vi "Daqmx Test VI.vi"() -> ()   [LabVIEW 2018]
uses:
  <vilib>/nisyscfg/Resource Expert Info.ctl
  <resource>/objmgr/daqmx.rc
  <vilib>/nisyscfg/nisyscfg.lvlib
  <resource>/objmgr/nicriosae.rc
panel:
  out "Array 3":string[](array[string])
  out "Array 2":string[](array[string])
  out "Experts":T1[][](array[typedef])
  out "Array":string[](array[string])
  out "Session out 2":refnum<k21> caption="Session out"
  out "Detected Systems":string[](array[string])
  out "DO.NumLines":u32
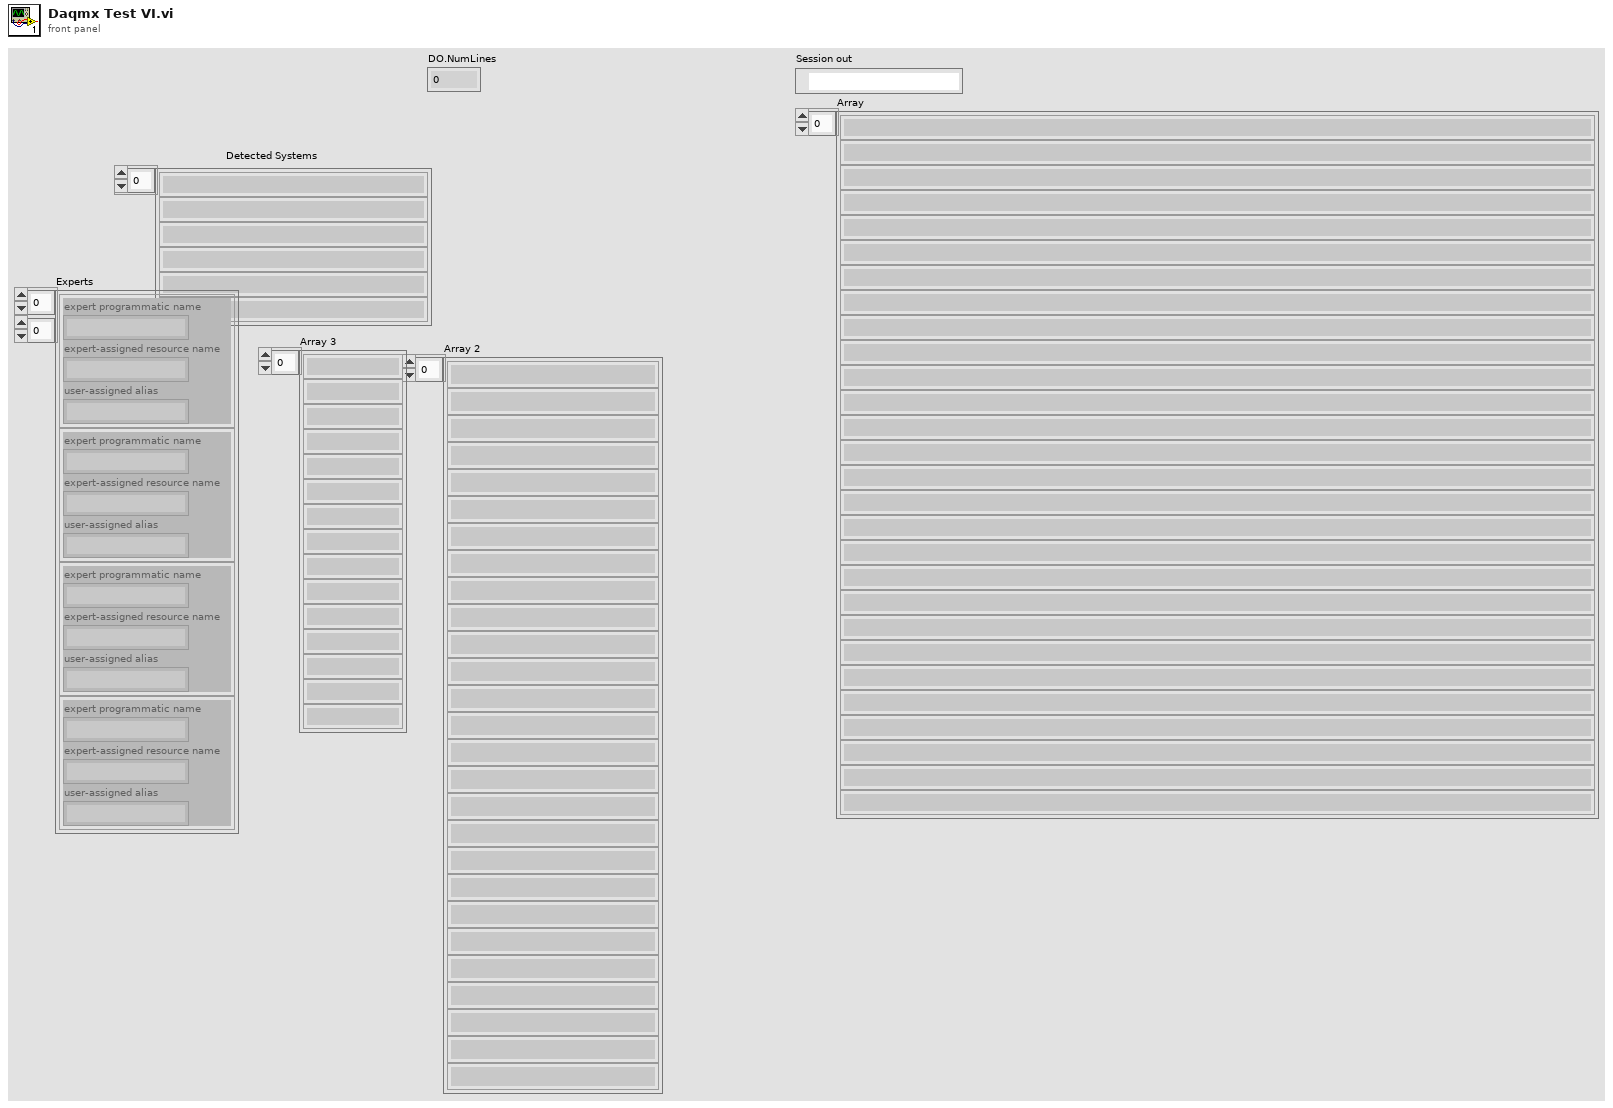
[diagram p1: front panel]
types:
  T1 = typedef "nisyscfg.lvlib/Resource Expert Info.ctl" = cluster{"expert programmatic name":string, "expert-assigned resource name":string, "user-assigned alias":string}
  T2 = typedef "Resource Expert Info.ctl" = cluster{"expert programmatic name":string, "expert-assigned resource name":string, "user-assigned alias":string}
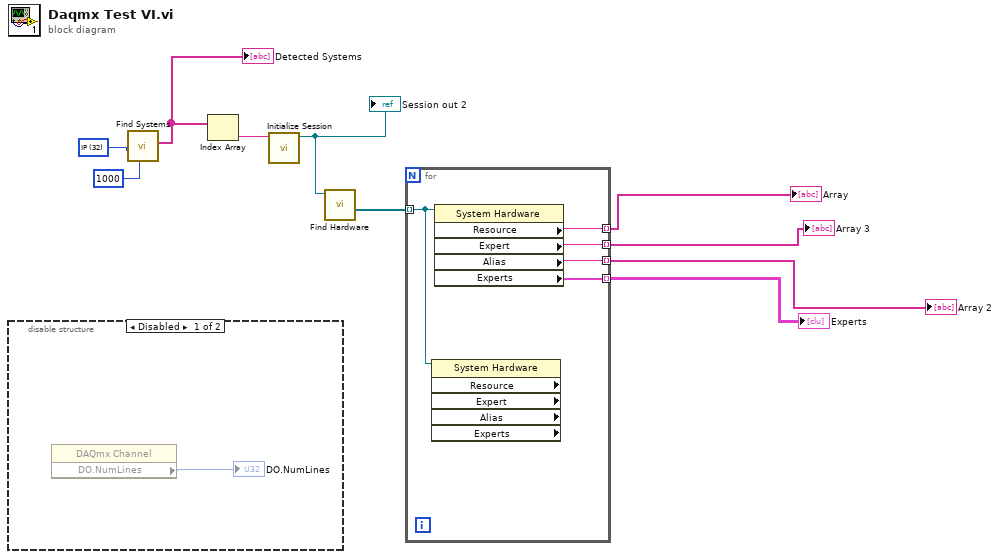
[diagram p0: block diagram]
diagram:
  w9 = u32 32 items=["Hostname"=16, "Hostname (IP)"=18, "Hostname (MAC)"=19, "IP"=32, "IP (Hostname)"=33, "IP (MAC)"=35, "MAC"=48, "MAC (Hostname)"=49, "MAC (IP)"=50] ("Output (Hostname and IP)")
  n1 = disable-structure shown="Disabled" {
    frame Disabled {
      n2 = property class="DAQmx Channel"() -> ("DO.NumLines"=→"DO.NumLines":u32)  [unwired: 2 in, 2 out]
    }
    frame Enabled {
    }
  }
  n3 = call <vilib>:"Find Systems.vi"("Timeout (4000 ms)"=u32 1000, "Output (Hostname and IP)"=w9) -> ("Detected Systems"=w8:string[])  [unwired: 7 in, 2 out]
  "Detected Systems" <- w8
  n4 = Index Array(array=w8) -> (element=w7:string)  [unwired: 1 in]
  n5 = call <vilib>:"Initialize Session.vi"("Target (localhost)"=w7) -> ("Session out"=w6:refnum<k21>)  [unwired: 9 in, 1 out]
  "Session out 2" <- w6
  n6 = call <vilib>:"Find Hardware.vi"("Session in"=w6) -> ("Resources out"=w5:refnum<k20>[])  [unwired: 7 in, 3 out]
  n7 = for {
    tunnel: w5 -> [w12] mode=indexing
    tunnel: [w16] -> w4 mode=indexing
    tunnel: [w15] -> w1 mode=indexing
    tunnel: [w14] -> w2 mode=indexing
    tunnel: [w13] -> w3 mode=indexing
    n8 = property class="System Hardware" props=["Resource", "Expert", "Alias", "Experts"](reference=w12) -> ()  [unwired: 1 in, 6 out]
    n9 = property class="System Hardware"(reference=w12) -> ("Resource"=w16:string, "Expert"=w15:string, "Alias"=w14:string, "Experts"=w13:T2[])  [unwired: 1 in, 2 out]
  }
  "Array" <- w4
  "Experts" <- w3
  "Array 2" <- w2
  "Array 3" <- w1
